vi "generateWaveform.vi"(8 "error in (no error)":errorcluster, 11 "SawtoothWave in":refnum<class "SawtoothWave.lvclass">) -> (0 "error out":errorcluster, 2 "Output":dbl, 3 "SawtoothWave out":refnum<class "SawtoothWave.lvclass">)   [LabVIEW 2015, in "SawtoothWave.lvclass"]
uses:
  SawtoothWave.lvclass
  SawtoothWave.lvclass/SawtoothWave.ctl
  <vilib>/ptbypt/NI_PtbyPt.lvlib
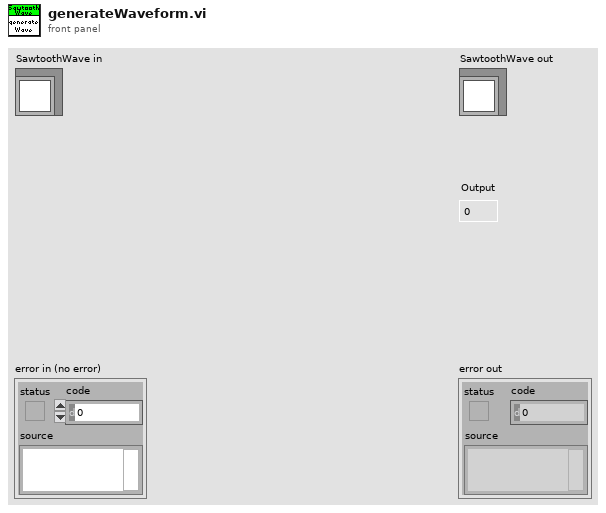
[diagram p1: front panel]
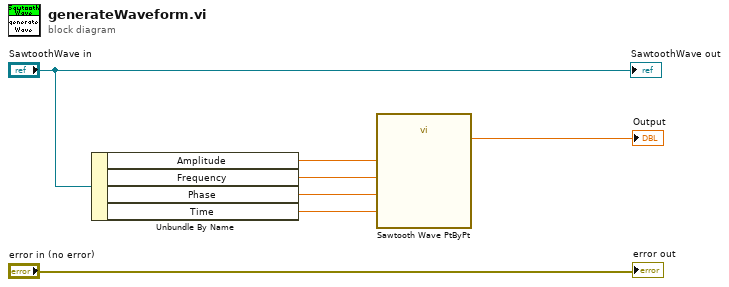
[diagram p0: block diagram]
diagram:
  n1 = Unbundle By Name("SawtoothWave in") -> ("Amplitude"=w6:dbl, "Frequency"=w5:dbl, "Phase"=w4:dbl, "Time"=w3:dbl)
  n2 = call <vilib>:"Sawtooth Wave PtByPt.vi"("time"=w3, "phase"=w4, "frequency"=w5, "amplitude"=w6) -> ("sawtooth wave"=→"Output":dbl)
  "error out" <- "error in (no error)"
  "SawtoothWave out" <- "SawtoothWave in"
